vi "MultiAxisPositioning.vi"(0 "connection ID":refnum<k5>, 5 "error in":errorcluster) -> (14 "connection ID":refnum<k5>, 19 "error out":errorcluster)   [LabVIEW 2016]
doc: "Simultaneously set 3 axes positions\n and get positions to minimize network latency"
panel:
  out "pos3":i32
  out "pos2":i32
  out "pos1":i32
  out "refpos3":i32
  out "refpos2":i32
  out "refpos1":i32
  out "ref3":bool
  out "ref2":bool
  out "ref1":bool
  in  "target3":i32
  in  "target2":i32
  in  "target1":i32
  in  "set3":bool
  in  "set2":bool
  in  "set1":bool
  out "params_cluster":T1
  in  "Params_cluster":T2
  in  "results_cluster":T3
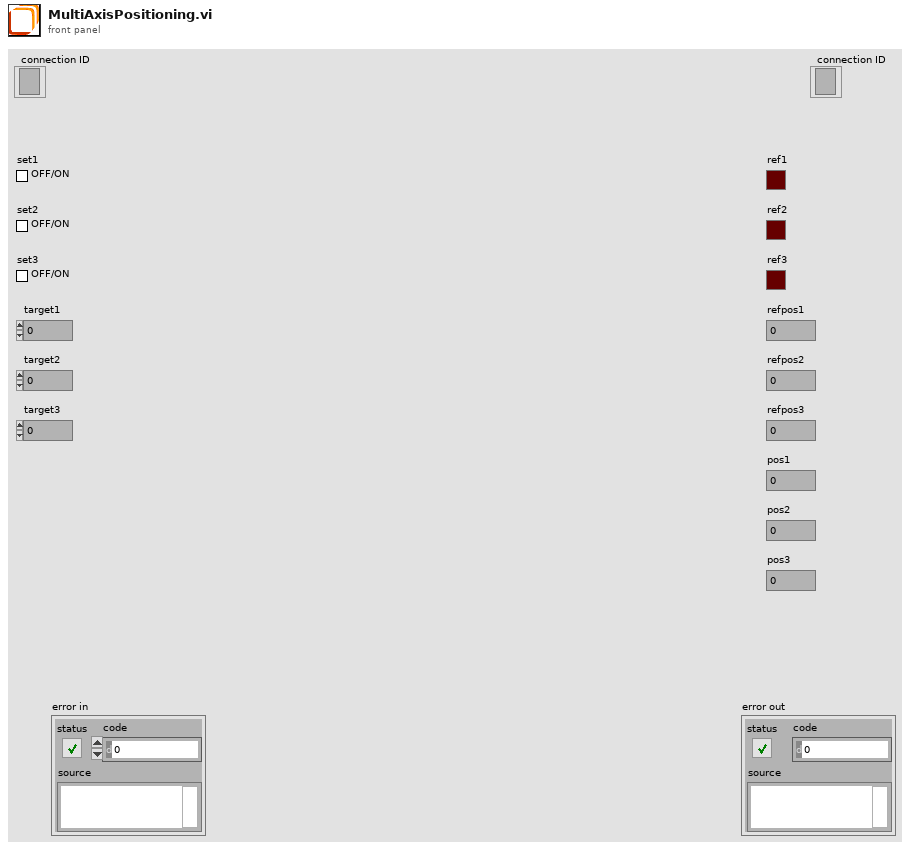
[diagram p1: front panel]
types:
  T1 = cluster{"set1":bool, "set2":bool, "set3":bool, "target1":i32, "target2":i32, "target3":i32}
  T2 = cluster{"boolean":bool, "boolean":bool, "boolean":bool, "integer":i32, "integer":i32, "integer":i32}
  T3 = cluster{"errNo":i32, "ref1":bool, "ref2":bool, "ref3":bool, "refpos1":i32, "refpos2":i32, "refpos3":i32, "pos1":i32, "pos2":i32, "pos3":i32}
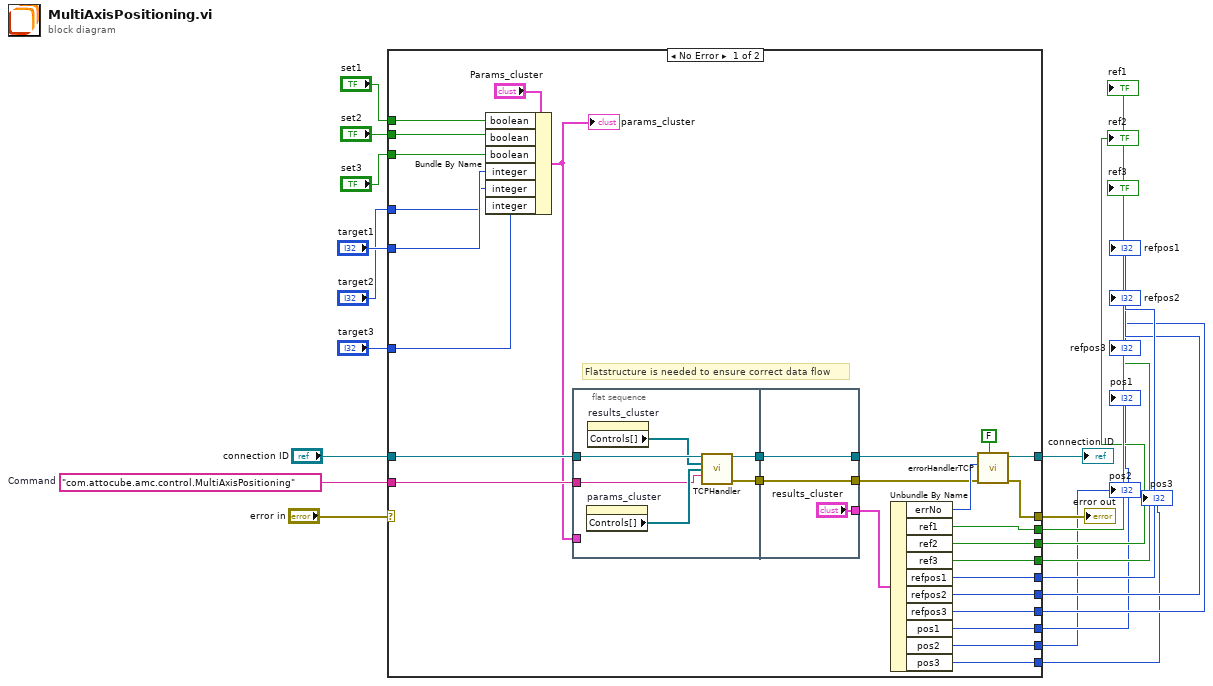
[diagram p0: block diagram]
diagram:
  w16 = "com.attocube.amc.control.MultiAxisPositioning"  # Command
  n1 = case shown="No Error" "error in" {
    selector: "error in" -> [_ w59]
    tunnel: [w46 w59] -> w20
    tunnel: [w48 w58] -> w19
    tunnel: "connection ID" -> [w45 w58]
    tunnel: w16 -> [w39 _]
    tunnel: "set1" -> [w35 _]
    tunnel: "set2" -> [w34 _]
    tunnel: "set3" -> [w33 _]
    tunnel: "target1" -> [w32 _]
    tunnel: "target2" -> [w31 _]
    tunnel: "target3" -> [w30 _]
    tunnel: [w29 _] -> w9
    tunnel: [w28 _] -> w8
    tunnel: [w27 _] -> w7
    tunnel: [w26 _] -> w6
    tunnel: [w25 _] -> w5
    tunnel: [w24 _] -> w4
    tunnel: [w23 _] -> w3
    tunnel: [w22 _] -> w2
    tunnel: [w21 _] -> w1
    frame No Error {
      # "Flatstructure is needed to ensure correct data flow"
      n2 = Bundle By Name(cluster="Params_cluster", "boolean"=w35, "boolean"=w34, "boolean"=w33, "integer"=w32, "integer"=w31, "integer"=w30) -> (w36:T2)
      "params_cluster" <- w36
      n3 = flat-sequence {
        tunnel: [w53] -> w41
        tunnel: w45 -> [w54]
        tunnel: w39 -> [w50]
        tunnel: [w49] -> w37
        tunnel: w36 -> [_]
        tunnel: ["results_cluster"] -> w42
        tunnel: [w57] -> w44
        tunnel: w41 -> [w57]
        tunnel: [w55] -> w38
        tunnel: w37 -> [w55]
        frame #0 {
          n4 = property on="params_cluster" class="Clust (strict)"() -> ("Controls[]"=w51:refnum<vi>[])  [unwired: 2 in, 2 out]
          n5 = property on="results_cluster" class="Clust (strict)"() -> ("Controls[]"=w52:refnum<vi>[])  [unwired: 2 in, 2 out]
          n6 = call "TCPHandler.vi"("connection ID"=w54, "results_cluster"=w52, "params_cluster"=w51, "method"=w50) -> ("connection ID"=w53:refnum<k5>, "error"=w49:errorcluster)  [unwired: 8 in, 2 out]
        }
        frame #1 {
        }
      }
      n7 = Unbundle By Name(w42) -> ("errNo"=w43:i32, "ref1"=w29:bool, "ref2"=w28:bool, "ref3"=w27:bool, "refpos1"=w26:i32, "refpos2"=w25:i32, "refpos3"=w24:i32, "pos1"=w23:i32, "pos2"=w22:i32, "pos3"=w21:i32)
      n8 = call "errorHandlerTCP.vi"("show popup"=FALSE, "error in"=w38, "error number"=w43, "connection ID"=w44) -> ("error out"=w46:errorcluster, "connection ID"=w48:refnum<k5>)  [unwired: 6 in]
    }
    frame Error {
    }
  }
  "error out" <- w20
  "connection ID" <- w19
  "ref1" <- w9
  "ref2" <- w8
  "ref3" <- w7
  "refpos1" <- w6
  "refpos2" <- w5
  "refpos3" <- w4
  "pos1" <- w3
  "pos2" <- w2
  "pos3" <- w1
